vi "Model Initial Values - Import RTM.vi"(8 "error in (no error)":errorcluster, 11 "Node Ptr":u64 format="%.0x") -> (0 "error out":errorcluster)   [LabVIEW 2011, in "Model Initial Values Custom Device.lvlib"]
uses:
  Model Initial Values Custom Device.lvlib
  Model Initial Values - Global.vi
  <vilib>/NI Veristand/Custom Device API/Set Item Property (String Array).vi
  <vilib>/NI Veristand/Custom Device API/Set Item Property (Double Array).vi
  <vilib>/NI Veristand/Custom Device Tools/Custom Device Utility Library/Custom Device Utility Library.lvlib
  <vilib>/NI Veristand/Custom Device API/Custom Device API.lvlib
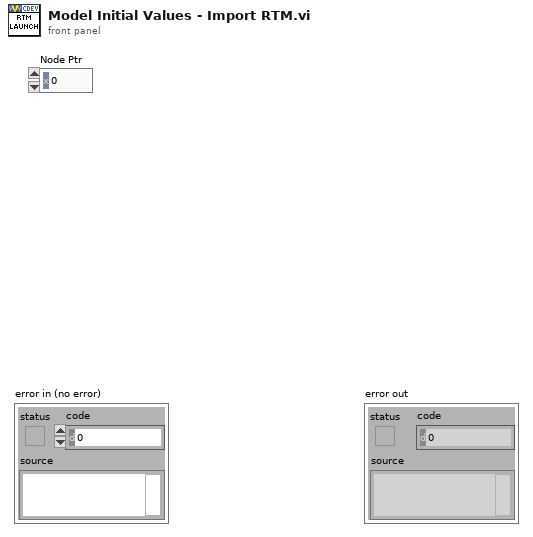
[diagram p1: front panel]
types:
  T1 = enum16{"open", "replace", "create", "open or create", "replace or create", "replace or create with confirmation"}
  T2 = typedef "Custom Device API.lvlib/Custom Device Item Ref.ctl" = u64
  T3 = cluster{"Name":string, "Is Channel":bool, "GUID":string}
  T4 = cluster{"Inport Refs":T2[], "Inport Names":string[], "Inport Default Values":dbl[]}
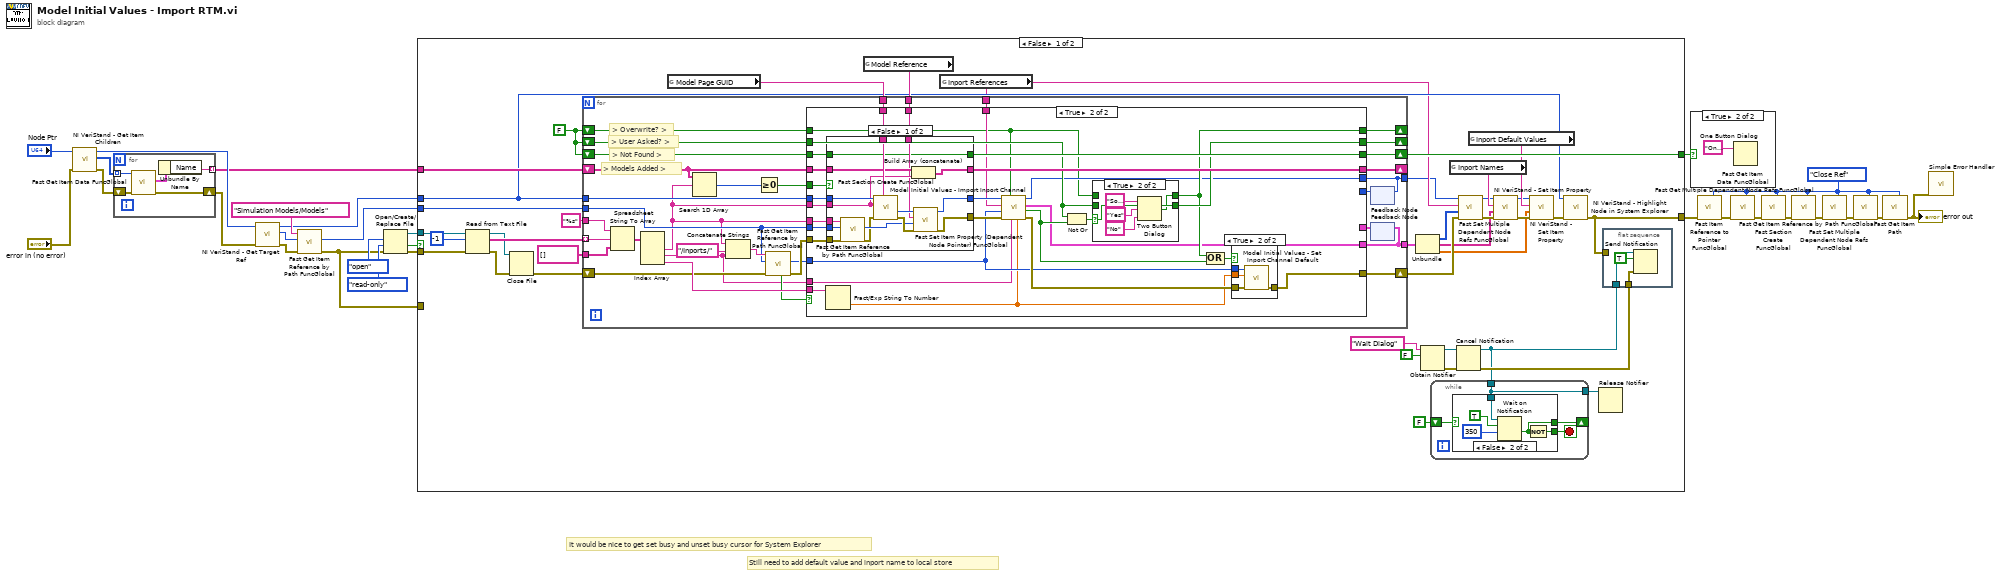
[diagram p0: block diagram]
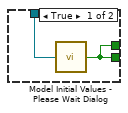
[diagram p3: hidden frame]
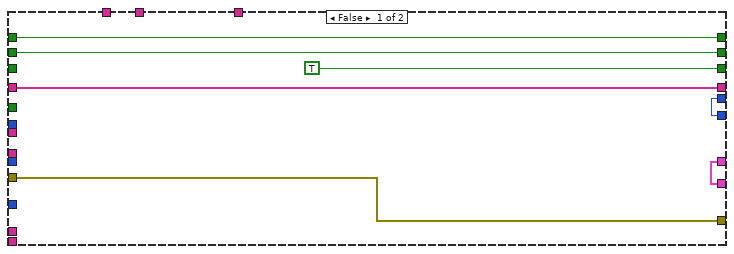
[diagram p4: hidden frame]
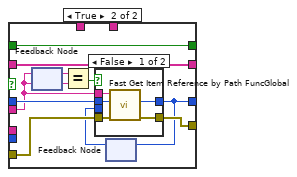
[diagram p7: hidden frame]
diagram:
  w2 = enum16{"Open or Add", "Close Ref"}."Close Ref" ("Action")
  # "Still need to add default value and inport name to local store"
  # "It would be nice to get set busy and unset busy cursor for System Explorer"
  n1 = call <vilib>:"NI VeriStand - Get Item Children.vi"("error in (no error)"="error in (no error)", "Item Ref in"="Node Ptr") -> ("error out"=w14:errorcluster, "Child Refs"=w16:T2[], "Item Ref out"=w18:T2)  [unwired: 6 in, 1 out]
  n2 = for {
    shift-right: [w31] -> w15
    shift-left: w14 -> [w32]
    tunnel: w16 -> [w29] mode=indexing
    tunnel: [w33] -> w13 mode=indexing
    n3 = call "Fast Get Item Data FuncGlobal.vi"("error in (no error)"=w32, "Item Ref in"=w29) -> ("error out"=w31:errorcluster, "Item Info"=w30:T3)  [unwired: 6 in, 2 out]
    n4 = Unbundle By Name(w30) -> ("Name"=w33:string)
  }
  n5 = call <vilib>:"NI VeriStand - Get Target Ref.vi"("error in"=w15, "Item Ref in"=w18) -> ("error out"=w24:errorcluster, "Target Ref"=w22:T2, "Item Ref out"=w20:T2)  [unwired: 6 in, 1 out]
  n6 = call "Fast Get Item Reference by Path FuncGlobal.vi"("error in (no error)"=w24, "Root Ref"=w22, "Item Path in"="Simulation Models/Models" ("Relative Item Path")) -> ("error out"=w1:errorcluster, "Item Ref"=w21:T2)  [unwired: 5 in, 2 out]
  n7 = Open/Create/Replace File(error in=w1, operation (0:open)=T1."open", access (0:read/write)=enum16{"read/write", "read-only", "write-only"}."read-only") -> (refnum out=w25:refnum<file>, cancelled=w12:bool, error out=w26:errorcluster)  [unwired: 3 in]
  n8 = case shown="False" w12 {
    tunnel: w26 -> [w55 _]
    tunnel: w25 -> [w72 _]
    tunnel: w21 -> [w67 _]
    tunnel: w20 -> [w58 _]
    tunnel: w13 -> [w64 _]
    tunnel: [w62 _] -> w11
    tunnel: [w34 w202] -> w5
    tunnel: w1 -> [_ w202]
    frame False {
      w66 = FALSE
      n9 = Read from Text File(file (use dialog)=w72, count=-1, error in=w55) -> (refnum out=w61:refnum<file>, text=w70:string[], error out=w60:errorcluster)  [unwired: 1 in, 1 out]
      n10 = Close File(refnum=w61, error in=w60) -> (error out=w59:errorcluster)  [unwired: 1 out]
      n11 = global read "Model Initial Values - Global.vi" "Model Page GUID"() -> (w65:string)
      n12 = global read "Model Initial Values - Global.vi" "Model Reference"() -> (w63:string)
      n13 = global read "Model Initial Values - Global.vi" "Inport References"() -> (w57:string)
      n14 = for {
        tunnel: w70 -> [w119] mode=indexing
        tunnel: "%s" ("format string") -> [w118]
        tunnel: string[] [] -> [w117]
        shift-right: [w99] -> _
        shift-left: w66 -> [w98]
        shift-right: [w100] -> _
        shift-left: w66 -> [w101]
        tunnel: w67 -> [w93]
        shift-right: [w107] -> w56
        shift-left: w59 -> [w94]
        shift-right: [w114] -> w62
        shift-left: w66 -> [w115]
        tunnel: w58 -> [w113]
        tunnel: w65 -> [w112]
        shift-right: [w106] -> _
        shift-left: w64 -> [w111]
        tunnel: w63 -> [w109]
        tunnel: w57 -> [w104]
        tunnel: [w91] -> w51
        tunnel: [w89] -> w54
        # "> Models Added >"
        # "> Not Found >"
        # "> Overwrite? >"
        # "> User Asked? >"
        n15 = Spreadsheet String To Array(format string=w118, spreadsheet string=w119, array type (2D Dbl)=w117) -> (array=w116:string[])  [unwired: 1 in]
        n16 = Index Array(array=w116) -> (element #1=w92:string, element #2=w87:string, element #3=w105:string)  [unwired: 3 in]
        n17 = Search 1D Array(1D array=w111, element=w92) -> (index of element=w110:i32)  [unwired: 1 in]
        n18 = Concatenate Strings(w92, "/Inports/" ("string"), w87) -> (w97:string)
        n19 = Greater Or Equal To 0?(x=w110) -> (x >= 0?=w108:bool)
        n20 = call "Fast Get Item Reference by Path FuncGlobal.vi"("error in (no error)"=w94, "Root Ref"=w93, "Item Path in"=w97) -> ("error out"=w103:errorcluster, "Item Ref"=w102:T2, "Found"=w95:bool)  [unwired: 5 in, 1 out]
        n21 = feedback #1() -> (w88:T2)  [unwired: 1 in]
        n22 = feedback #2() -> (w90:T4)  [unwired: 1 in]
        n23 = case shown="True" w95 {
          tunnel: w115 -> [_ w156]
          tunnel: [TRUE w155] -> w114
          tunnel: w113 -> [_ w154]
          tunnel: w112 -> [_ w153]
          tunnel: w111 -> [w124 w152]
          tunnel: w92 -> [_ w151]
          tunnel: w109 -> [_ w150]
          tunnel: w103 -> [w125 w149]
          tunnel: w93 -> [_ w145]
          tunnel: w108 -> [_ w148]
          tunnel: [w125 w135] -> w107
          tunnel: [w124 w147] -> w106
          tunnel: w105 -> [_ w144]
          tunnel: w104 -> [_ w134]
          tunnel: w102 -> [_ w136]
          tunnel: w101 -> [w122 w140]
          tunnel: [w122 w141] -> w100
          tunnel: [w123 w139] -> w99
          tunnel: w98 -> [w123 w127]
          tunnel: w92 -> [_ w132]
          tunnel: [w121 w131] -> w91
          tunnel: w90 -> [w121 _]
          tunnel: [w120 w130] -> w89
          tunnel: w88 -> [w120 _]
          tunnel: w87 -> [_ w129]
          frame False {
          }
          frame True {
            n24 = Fract/Exp String To Number(string=w144) -> (number=w128:dbl)  [unwired: 3 in, 1 out]
            n25 = case shown="False" w148 {
              tunnel: w156 -> [w176 w194]
              tunnel: [w176 w194] -> w155
              tunnel: w154 -> [w184 w192]
              tunnel: w153 -> [w183 _]
              tunnel: w151 -> [w181 w188]
              tunnel: w149 -> [w172 w191]
              tunnel: w145 -> [w170 _]
              tunnel: w152 -> [w182 w193]
              tunnel: [w180 w193] -> w147
              tunnel: w150 -> [w177 _]
              tunnel: [w175 w186] -> w146
              tunnel: [w174 w190] -> w143
              tunnel: w132 -> [w169 _]
              frame False {
                n26 = call "Fast Get Item Reference by Path FuncGlobal.vi"("error in (no error)"=w172, "Root Ref"=w170, "Item Path in"=w169) -> ("error out"=w171:errorcluster, "Item Ref"=w173:T2)  [unwired: 5 in, 2 out]
                n27 = call "Fast Section Create FuncGlobal.vi"("GUID (Default Section)"=w183, "error in (no error)"=w171, "Section Name"=w181, "Parent Ref in"=w184) -> ("error out"=w178:errorcluster, "Section Ptr"=w179:T2)  [unwired: 4 in, 2 out]
                n28 = Build Array (concatenate)(w182, w181) -> (w180:string[])
                n29 = call "Fast Set Item Property (Dependent Node Pointer) FuncGlobal.vi"("error in (no error)"=w178, "Dependent Node Ref"=w173, "Property Name"=w177, "Item Ref in"=w179) -> ("error out"=w174:errorcluster, "Item Ref out"=w175:T2)  [unwired: 5 in, 1 out]
              }
              frame True {
                n30 = feedback-in #3(w188) -> ()
                n31 = feedback #3() -> (w189:string)  [unwired: 1 in]
                n32 = Equal?(x=w189, y=w188) -> (x = y?=w187:bool)
                n33 = feedback #4() -> (w185:T2)  [unwired: 1 in]
                n34 = case shown="False" w187 {
                  tunnel: w192 -> [w199 _]
                  tunnel: w191 -> [w198 w201]
                  tunnel: [w197 w200] -> w186
                  tunnel: [w196 w201] -> w190
                  tunnel: w188 -> [w195 _]
                  tunnel: w185 -> [_ w200]
                  frame False {
                    n35 = call "Fast Get Item Reference by Path FuncGlobal.vi"("error in (no error)"=w198, "Root Ref"=w199, "Item Path in"=w195) -> ("error out"=w196:errorcluster, "Item Ref"=w197:T2)  [unwired: 5 in, 2 out]
                  }
                  frame True {
                  }
                }
                n36 = feedback-in #4(w186) -> ()
              }
            }
            n37 = call "Model Initial Values - Import Inport Channel.vi"("Initial Value"=w128, "Inport Name"=w129, "Overwrite?"=w127, "error in"=w143, "Inport Ref"=w136, "Inport References"=w134, "Section Ref"=w146) -> ("error out"=w138:errorcluster, "Created New?"=w133:bool, "Dependent Nodes"=w131:T4, "Section Ref out"=w130:T2)  [unwired: 1 in]
            n38 = Not Or(1:w133, 2:w140) -> (0:w142:bool)
            n39 = case shown="True" w142 {
              selector: w142 -> [_ w165]
              tunnel: [w163 w165] -> w141
              tunnel: w140 -> [w163 _]
              tunnel: [w162 w164] -> w139
              tunnel: w127 -> [w162 _]
              frame False {
              }
              frame True {
                n40 = Two Button Dialog(message="Some of the Inports already exist. Would you like to overwrite?", 1:"No" ("F button name (\"Cancel\")"), 2:"Yes" ("T button name (\"OK\")")) -> (T button?=w164:bool)
              }
            }
            n41 = Compound Arithmetic op=OR(w139, w133) -> (w137:bool)
            n42 = case shown="True" w137 {
              tunnel: w136 -> [_ w161]
              tunnel: w128 -> [_ w160]
              tunnel: w138 -> [w157 w159]
              tunnel: [w157 w158] -> w135
              frame False {
              }
              frame True {
                n43 = call "Model Initial Values - Set Inport Channel Default.vi"("error in"=w159, "Default Value"=w160, "Item Ref in"=w161) -> ("error out"=w158:errorcluster)  [unwired: 7 in, 1 out]
              }
            }
          }
        }
        n44 = feedback-in #1(w89) -> ()
        n45 = feedback-in #2(w91) -> ()
      }
      n46 = Unbundle(w51) -> ("Inport Refs"=w50:T2[], "Inport Names"=w48:string[], "Inport Default Values"=w43:dbl[])
      n47 = Obtain Notifier(name (unnamed)="Wait Dialog", notification data type=FALSE) -> (notifier out=w40:refnum<notifier>, error out=w37:errorcluster)  [unwired: 2 in, 1 out]
      n48 = global read "Model Initial Values - Global.vi" "Inport Names"() -> (w52:string)
      n49 = Cancel Notification(0:w40, 3:w37) -> (8:w35:refnum<notifier>, 11:w36:errorcluster)  [unwired: 1 out]
      n50 = while {
        tunnel: w35 -> [w73]
        shift-right: [w74] -> _
        shift-left: FALSE -> [w75]
        tunnel: [w73] -> w38
        stop <- w76 stop-if-true
        n51 = case shown="False" w75 {
          tunnel: [w77 w81] -> w76
          tunnel: w73 -> [w78 w83]
          tunnel: [w77 w79] -> w74
          frame True {
            n52 = call "Model Initial Values - Please Wait Dialog.vi"("notifier out"=w78) -> ("Boolean"=w77:bool)
          }
          frame False {
            n53 = Wait on Notification(notifier=w83, ignore previous (F)=TRUE, timeout in ms (-1)=350) -> (timed out?=w79:bool)  [unwired: 1 in, 3 out]
            n54 = Not(x=w79) -> (.not. x?=w81:bool)
          }
        }
      }
      n55 = call "Fast Set Multiple Dependent Node Refs FuncGlobal.vi"("error in (no error)"=w56, "Dependent Node Refs"=w50, "Base Property Name"=w57, "Item Ref in"=w54) -> ("error out"=w53:errorcluster, "Item Ref out"=w49:T2)  [unwired: 6 in]
      n56 = global read "Model Initial Values - Global.vi" "Inport Default Values"() -> (w45:string)
      n57 = call-poly <vilib>:"NI VeriStand - Set Item Property.vi"("error in (no error)"=w53, "Value"=w48, "Property Name"=w52, "Item Ref in"=w49) -> ("error out"=w47:errorcluster, "Item Ref out"=w44:T2)  [unwired: 5 in, 1 out]
      n58 = call-poly <vilib>:"NI VeriStand - Set Item Property.vi"("error in (no error)"=w47, "Value"=w43, "Property Name"=w45, "Item Ref in"=w44) -> ("error out"=w46:errorcluster)  [unwired: 5 in, 2 out]
      n59 = call <vilib>:"NI VeriStand - Highlight Node in System Explorer.vi"("error in (no error)"=w46, "Item Ref in"=w58) -> ("error out"=w34:errorcluster)  [unwired: 8 in, 1 out]
      n60 = Release Notifier(notifier=w38) -> ()  [unwired: 2 in, 3 out]
      n61 = flat-sequence {
        tunnel: w35 -> [w86]
        tunnel: w36 -> [w85]
        tunnel: w34 -> [_]
        frame #0 {
          n62 = Send Notification(notification=TRUE, notifier=w86, error in (no error)=w85) -> ()  [unwired: 2 out]
        }
      }
    }
    frame True {
    }
  }
  n63 = case shown="True" w11 {
    frame False {
    }
    frame True {
      n64 = One Button Dialog(message="One or more models and/or inports were not found in the system definition and therefore were not imported.") -> ()  [unwired: 1 in, 1 out]
    }
  }
  n65 = call "Fast Item Reference to Pointer FuncGlobal.vi"("Action"=w2, "error in (no error)"=w5) -> ("error out"=w10:errorcluster)  [unwired: 6 in, 3 out]
  n66 = call "Fast Get Item Data FuncGlobal.vi"("Action"=w2, "error in (no error)"=w10) -> ("error out"=w7:errorcluster)  [unwired: 6 in, 3 out]
  n67 = call "Fast Section Create FuncGlobal.vi"("Action"=w2, "error in (no error)"=w7) -> ("error out"=w8:errorcluster)  [unwired: 6 in, 3 out]
  n68 = call "Fast Get Multiple Dependent Node Refs FuncGlobal.vi"("Action"=w2, "error in (no error)"=w8) -> ("error out"=w9:errorcluster)  [unwired: 7 in, 2 out]
  n69 = call "Fast Set Multiple Dependent Node Refs FuncGlobal.vi"("Action"=w2, "error in (no error)"=w9) -> ("error out"=w6:errorcluster)  [unwired: 8 in, 1 out]
  n70 = call "Fast Get Item Reference by Path FuncGlobal.vi"("Action"=w2, "error in (no error)"=w6) -> ("error out"=w4:errorcluster)  [unwired: 6 in, 3 out]
  n71 = call "Fast Get Item Path.vi"("Action"=w2, "error in (no error)"=w4) -> ("error out"=w3:errorcluster)  [unwired: 6 in, 3 out]
  "error out" <- w3
  n72 = call <vilib>:"Simple Error Handler.vi"("error in (no error)"=w3) -> ()  [unwired: 4 in, 5 out]
